vi "ScopeTakeMeasurement.vi"(10 "Scope Error":errorcluster, 11 "Scope VISA":refnum<visa-resource-name>) -> (0 "dt":dbl, 1 "Data":dbl[](array[numeric]), 2 "error out":errorcluster, 3 "VISA resource name out":refnum<visa-resource-name>)   [LabVIEW 2021]
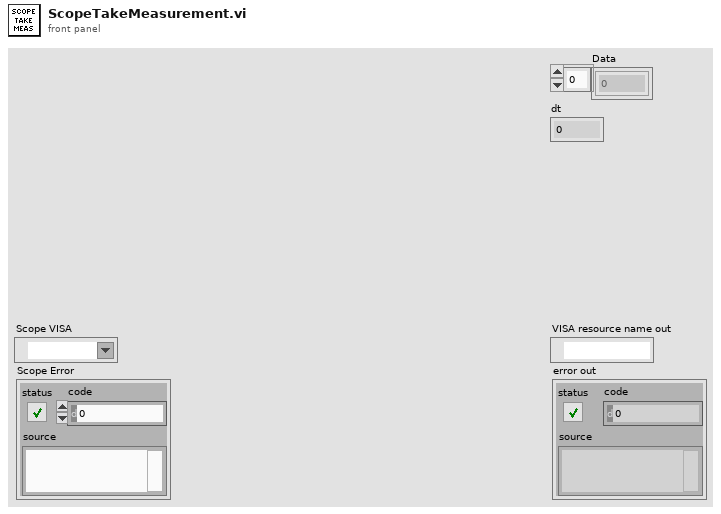
[diagram p1: front panel]
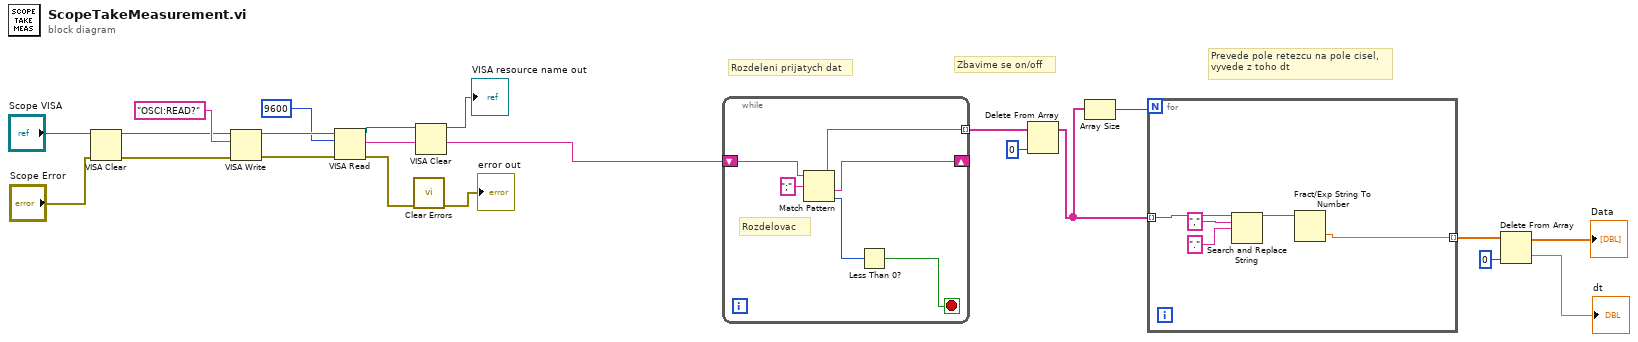
[diagram p0: block diagram]
diagram:
  # "Zbavime se on/off"
  # "Rozdeleni prijatych dat"
  # "Prevede pole retezcu na pole cisel,\nvyvede z toho dt"
  n1 = VISA Clear(VISA resource name="Scope VISA", error in (no error)="Scope Error") -> (VISA resource name out=w3:refnum<visa-resource-name>, error out=w1:errorcluster)
  n2 = VISA Write(VISA resource name=w3, write buffer="OSCI:READ?", error in (no error)=w1) -> (VISA resource name out=w19:refnum<visa-resource-name>, error out=w18:errorcluster)  [unwired: 1 out]
  n3 = VISA Read(VISA resource name=w19, byte count=u32 9600, error in (no error)=w18) -> (VISA resource name out=w13:refnum<visa-resource-name>, read buffer=w16:string, error out=w15:errorcluster)  [unwired: 1 out]
  n4 = call <vilib>:"Clear Errors.vi"("error in (no error)"=w15) -> ("error out"=→"error out":errorcluster)  [unwired: 5 in, 1 out]
  n5 = VISA Clear(VISA resource name=w13) -> (VISA resource name out=→"VISA resource name out":refnum<visa-resource-name>)  [unwired: 1 in, 1 out]
  n6 = while {
    shift-right: [w23] -> _
    shift-left: w16 -> [w24]
    tunnel: [w22] -> w12 mode=indexing
    stop <- w25 stop-if-true
    # "Rozdelovac"
    n7 = Match Pattern(string=w24, regular expression=";") -> (before substring=w22:string, after substring=w23:string, offset past match=w26:i32)  [unwired: 1 in, 1 out]
    n8 = Less Than 0?(x=w26) -> (x < 0?=w25:bool)
  }
  n9 = Delete From Array(array=w12, index=0) -> (array with subset deleted=w10:string[])  [unwired: 1 in, 1 out]
  n10 = Array Size(array=w10) -> (size(s)=w9:i32)
  n11 = for {
    N: w9 -> [_]
    tunnel: w10 -> [w31] mode=indexing
    tunnel: [w32] -> w8 mode=indexing
    n12 = Search and Replace String(input string=w31, search string=",", replace string="." ("replace string (\"\")")) -> (result string=w28:string)  [unwired: 5 in, 3 out]
    n13 = Fract/Exp String To Number(string=w28) -> (number=w32:dbl)  [unwired: 3 in, 1 out]
  }
  n14 = Delete From Array(array=w8, index=0) -> (deleted portion=→"dt":dbl, array with subset deleted=→"Data":dbl[])  [unwired: 1 in]
